vi "GetInstrumentHandle.vi"(8 "error in (no error)":errorcluster, 11 "AnalogDiscoveryFunction in":refnum<class "AnalogDiscoveryFunction.lvclass">) -> (0 "error out":errorcluster, 2 "Instrument Handle":u32, 3 "AnalogDiscoveryFunction out":refnum<class "AnalogDiscoveryFunction.lvclass">)   [LabVIEW 2020, in "AnalogDiscoveryFunction.lvclass"]
uses:
  AnalogDiscoveryFunction.lvclass
  AnalogDiscoveryFunction.lvclass/AnalogDiscoveryFunction.ctl
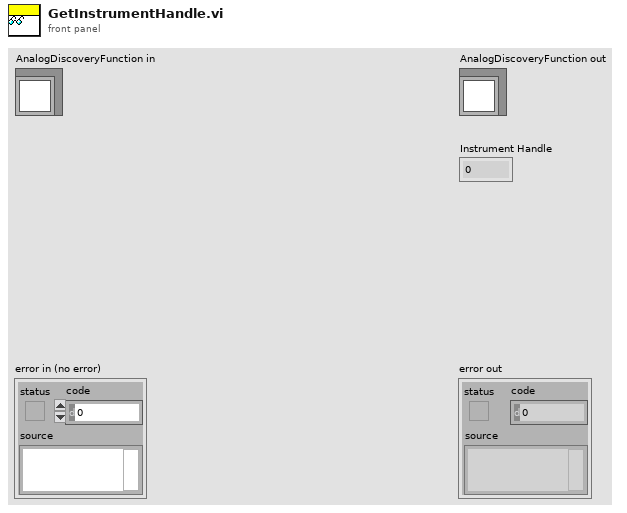
[diagram p1: front panel]
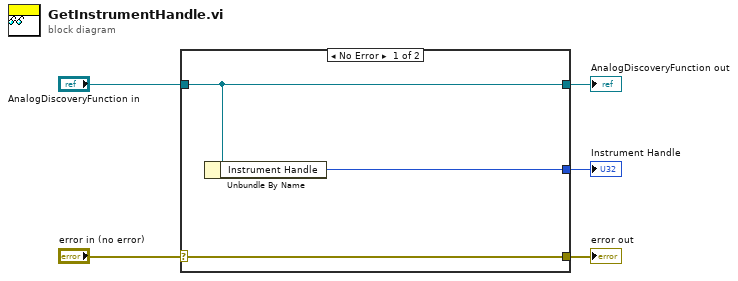
[diagram p0: block diagram]
diagram:
  n1 = case shown="No Error" "error in (no error)" {
    selector: "error in (no error)" -> [w8 w9]
    tunnel: [w8 w9] -> w4
    tunnel: [w7 w10] -> w2
    tunnel: "AnalogDiscoveryFunction in" -> [w7 w10]
    tunnel: [w6 _] -> w1
    frame No Error {
      n2 = Unbundle By Name(w7) -> ("Instrument Handle"=w6:u32)
    }
    frame Error {
    }
  }
  "error out" <- w4
  "AnalogDiscoveryFunction out" <- w2
  "Instrument Handle" <- w1
